vi "NI VeriStand - Get Macro Recorder Command Lines.vi"(8 "error in (no error)":errorcluster, 11 "MacroRecorder in":T3) -> (0 "error out":errorcluster, 2 "Command Lines":T1, 3 "MacroRecorder out":T3)   [LabVIEW 2020, in "NI_VS MacroRecorderAPI.lvlib"]
doc: "Returns the commands the VeriStand Gateway sends to the RT target or desktop PC. You must use the Open Command Line Notification (Macro Recorder) VI to open a reference to the command line of the Macro Recorder tool before you call this VI."
uses:
  <vilib>/NI VeriStand/Execution/MacroRecorder/NI_VS MacroRecorderAPI.lvlib
  <vilib>/NI VeriStand/Execution/MacroRecorder/MacroRecorderAPI.ctl
  NationalInstruments.VeriStand.ClientAPI
  <vilib>/NI VeriStand/Execution/MacroRecorder/Command Lines.ctl
  <vilib>/NI VeriStand/Execution/MacroRecorder/Command Line Info.ctl
  NationalInstruments.VeriStand.WorkspaceMacro
  <vilib>/NI VeriStand/Execution/MacroPlayer/Command Line Info.ctl
  <vilib>/NI VeriStand/Execution/MacroPlayer/NI_VS MacroPlayerAPI.lvlib
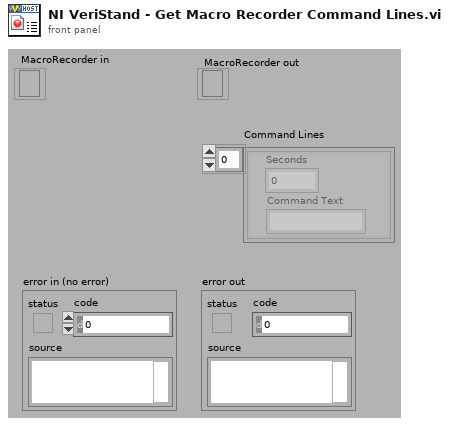
[diagram p1: front panel]
types:
  T1 = typedef "NI_VS MacroRecorderAPI.lvlib/Command Lines.ctl" = T2[]
  T2 = typedef "NI_VS MacroRecorderAPI.lvlib/Command Line Info.ctl" = cluster{"Seconds":dbl, "Command Text":string}
  T3 = typedef "NI_VS MacroRecorderAPI.lvlib/MacroRecorderAPI.ctl" = refnum<k24>
  T4 = typedef "NI_VS MacroPlayerAPI.lvlib/Command Line Info.ctl" = cluster{"Seconds":dbl, "Command Text":string}
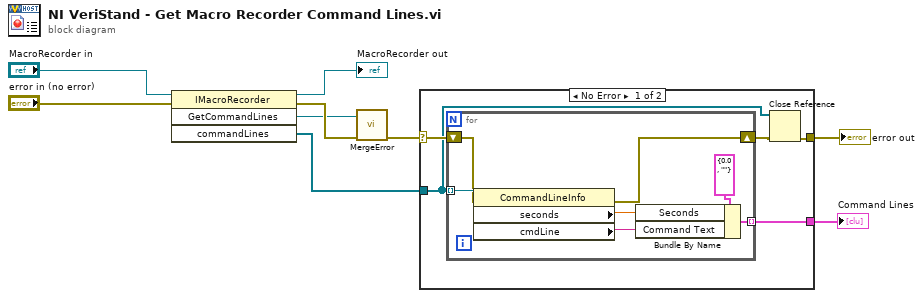
[diagram p0: block diagram]
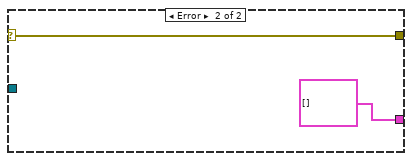
[diagram p2: hidden frame]
diagram:
  n1 = invoke class="IMacroRecorder" method="GetCommandLines"(reference="MacroRecorder in", error in="error in (no error)") -> (reference out=→"MacroRecorder out":T3, error out=w7:errorcluster, "GetCommandLines"=w5:refnum<k24>, "commandLines"=w3:refnum<k24>[])  [unwired: 2 in]
  n2 = call <vilib>:"MergeError.vi"("error in (no error)"=w7, "Error"=w5) -> ("error out"=w4:errorcluster)  [unwired: 9 out]
  n3 = case shown="No Error" w4 {
    selector: w4 -> [w13 w22]
    tunnel: [w14 T4[] []] -> w2
    tunnel: w3 -> [w10 _]
    tunnel: [w11 w22] -> w1
    frame No Error {
      n4 = for {
        tunnel: w10 -> [w21] mode=indexing
        tunnel: [w17] -> w14 mode=indexing
        shift-right: [w15] -> w12
        shift-left: w13 -> [w16]
        n5 = property class="CommandLineInfo"(reference=w21, error in=w16) -> (error out=w15:errorcluster, "seconds"=w19:dbl, "cmdLine"=w18:string)  [unwired: 1 out]
        n6 = Bundle By Name(cluster=T2 {"Seconds"=0.0, "Command Text"=""} ("Macro Table Info"), "Seconds"=w19, "Command Text"=w18) -> (w17:T2)
      }
      n7 = Close Reference(reference=w10, error in (no error)=w12) -> (error out=w11:errorcluster)
    }
    frame Error {
    }
  }
  "error out" <- w1
  "Command Lines" <- w2
